vi "日志、报警信息存储 (子VI).vi"() -> ()   [LabVIEW 2016, in "德润DR803L超标留样.lvlib"]
panel:
  out "采样器状态":T1
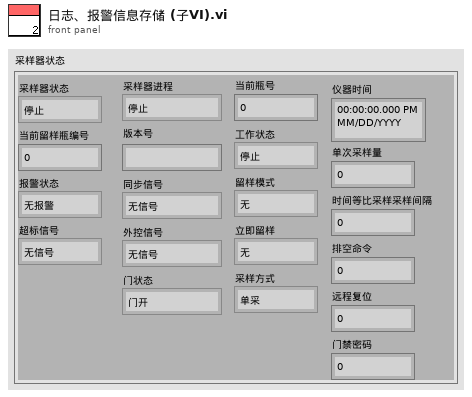
[diagram p1: front panel]
types:
  T1 = cluster{"采样器状态":enum16{"停止", "运行"}, "当前留样瓶编号":u16, "报警状态":enum16{"无报警", "缺水报警"}, "超标信号":enum16{"无信号", "超标信号"}, "采样器进程":enum16{"停止", "待机", "定位校正", "移除瓶盖", "采样瓶排空", "管路润洗", "管存", "进样", "瓶盖密封", "管路排空", "调整采样位置", "采样结束", "采样瓶润洗", "瓶润洗排空"}, "版本号":string, "同步信号":enum16{"无信号", "同步信号"}, "外控信号":enum16{"无信号", "外控信号"}, "门状态":enum16{"门开", "门关"}, "当前瓶号":u16, "工作状态":enum16{"停止", "采样中"}, "留样模式":enum16{"无", "定时留样", "时间等比例", "超标留样", "同步留样", "外控留样"}, "立即留样":enum16{"无", "远程留样"}, "采样方式":enum16{"单采", "双重"}, "仪器时间":timestamp, "单次采样量":u16, "时间等比采样采样间隔":u16, "排空命令":u16, "远程复位":u16, "门禁密码":u16}
  T2 = cluster{"时间标识":timestamp, "设备":string, "日志信息":string, "流程参数":string}
  T3 = cluster{"时间标识":timestamp, "设备":string, "日志信息":string}
  T4 = enum16{"停止", "待机", "定位校正", "移除瓶盖", "采样瓶排空", "管路润洗", "管存", "进样", "瓶盖密封", "管路排空", "调整采样位置", "采样结束", "采样瓶润洗", "瓶润洗排空"}
  T5 = enum16{"无", "定时留样", "时间等比例", "超标留样", "同步留样", "外控留样"}
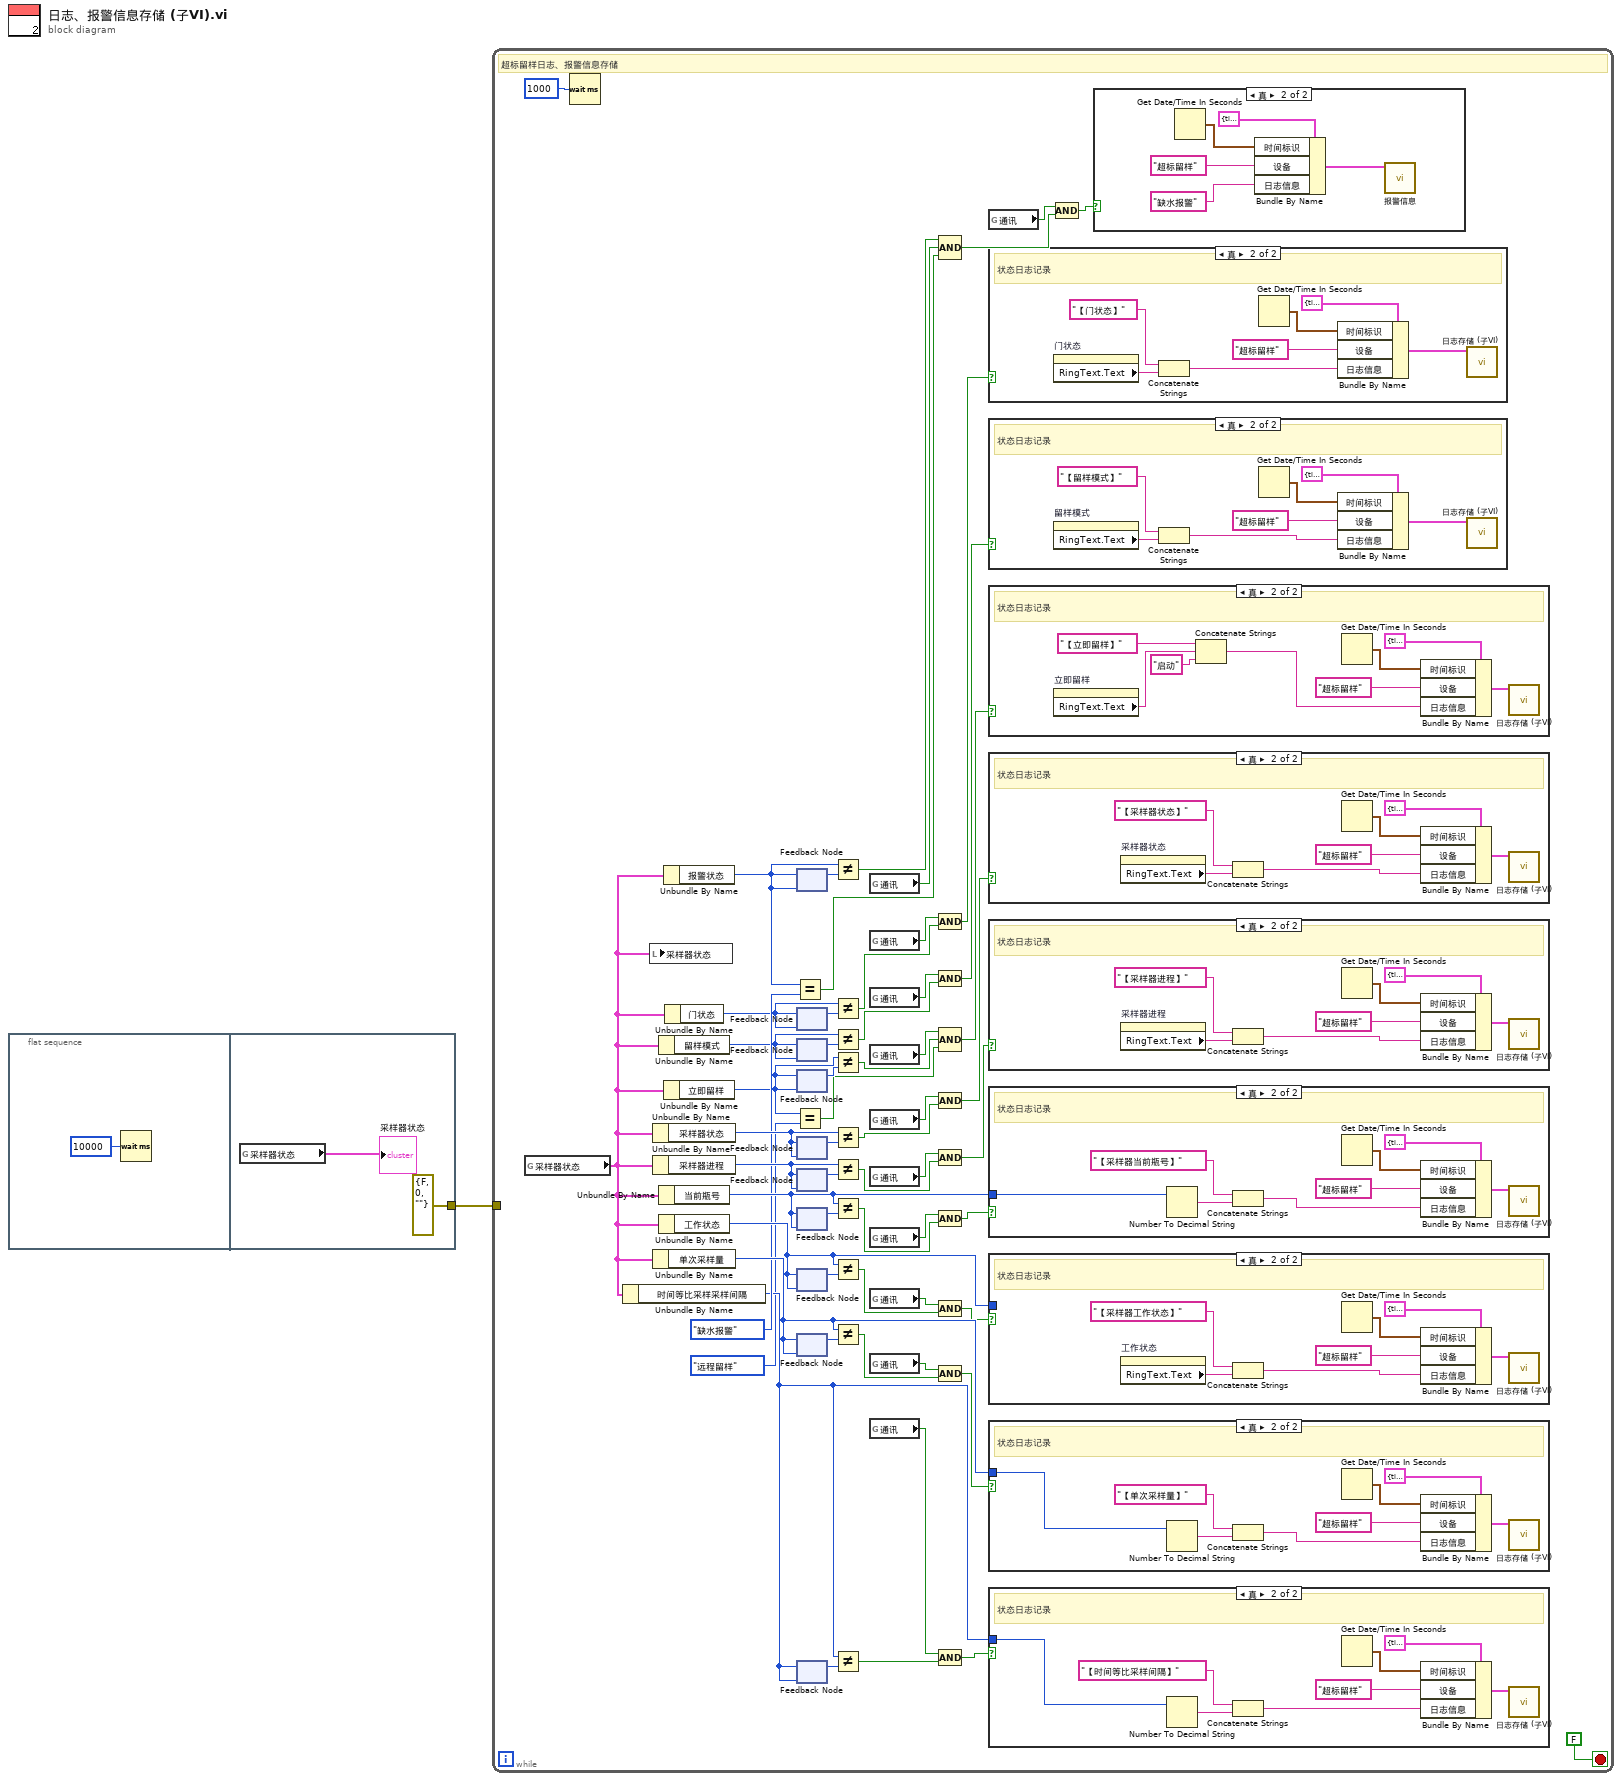
[diagram p0: block diagram]
diagram:
  n1 = flat-sequence {
    tunnel: [errorcluster {"status"=FALSE, "code"=0, "source"=""} ("错误常量")] -> w1
    frame #0 {
      n2 = Wait (ms)(milliseconds to wait=u32 10000 ("等待时间（毫秒）")) -> ()  [unwired: 1 out]
    }
    frame #1 {
      n3 = global read "超标留样全局.vi" "采样器状态"() -> (→"采样器状态":T1)
    }
  }
  n4 = while {
    tunnel: w1 -> [_]
    stop <- FALSE stop-if-true
    # "超标留样日志、报警信息存储"
    n5 = global read "超标留样全局.vi" "采样器状态"() -> (w5:T1)
    n6 = Wait (ms)(milliseconds to wait=u32 1000 ("等待时间（毫秒）")) -> ()  [unwired: 1 out]
    n7 = Unbundle By Name(w5) -> ("时间等比采样采样间隔"=w41:u16)
    n8 = local write "采样器状态"(w5) -> ()
    n9 = Unbundle By Name(w5) -> ("采样器状态"=w60:enum16{"停止", "运行"})
    n10 = Unbundle By Name(w5) -> ("采样器进程"=w59:T4)
    n11 = Unbundle By Name(w5) -> ("单次采样量"=w52:u16)
    n12 = Unbundle By Name(w5) -> ("留样模式"=w44:T5)
    n13 = Unbundle By Name(w5) -> ("当前瓶号"=w56:u16)
    n14 = Unbundle By Name(w5) -> ("工作状态"=w55:enum16{"停止", "采样中"})
    n15 = Unbundle By Name(w5) -> ("报警状态"=w47:enum16{"无报警", "缺水报警"})
    n16 = Unbundle By Name(w5) -> ("立即留样"=w40:enum16{"无", "远程留样"})
    n17 = Unbundle By Name(w5) -> ("门状态"=w45:enum16{"门开", "门关"})
    n18 = Equal?(x=w47, y=enum16{"无报警", "缺水报警"}."缺水报警" ("报警状态")) -> (x = y?=w35:bool)
    n19 = Equal?(x=w40, y=enum16{"无", "远程留样"}."远程留样" ("立即留样")) -> (x = y?=w8:bool)
    n20 = feedback #1(w47) -> (w50:enum16{"无报警", "缺水报警"})
    n21 = feedback-in #1(w47) -> ()
    n22 = feedback #2(w45) -> (w46:enum16{"门开", "门关"})
    n23 = feedback-in #2(w45) -> ()
    n24 = feedback #3(w44) -> (w43:T5)
    n25 = feedback-in #3(w44) -> ()
    n26 = feedback #4(w40) -> (w39:enum16{"无", "远程留样"})
    n27 = feedback-in #4(w40) -> ()
    n28 = feedback #5(w60) -> (w61:enum16{"停止", "运行"})
    n29 = feedback-in #5(w60) -> ()
    n30 = feedback #6(w59) -> (w58:T4)
    n31 = feedback-in #6(w59) -> ()
    n32 = feedback #7(w56) -> (w57:u16)
    n33 = feedback-in #7(w56) -> ()
    n34 = feedback #8(w55) -> (w54:enum16{"停止", "采样中"})
    n35 = feedback-in #8(w55) -> ()
    n36 = feedback #9(w52) -> (w53:u16)
    n37 = feedback-in #9(w52) -> ()
    n38 = feedback #10(w41) -> (w42:u16)
    n39 = feedback-in #10(w41) -> ()
    n40 = Not Equal?(x=w47, y=w50) -> (x != y?=w34:bool)
    n41 = Not Equal?(x=w45, y=w46) -> (x != y?=w31:bool)
    n42 = Not Equal?(x=w44, y=w43) -> (x != y?=w23:bool)
    n43 = Not Equal?(x=w40, y=w39) -> (x != y?=w7:bool)
    n44 = Not Equal?(x=w60, y=w61) -> (x != y?=w25:bool)
    n45 = Not Equal?(x=w59, y=w58) -> (x != y?=w26:bool)
    n46 = Not Equal?(x=w56, y=w57) -> (x != y?=w19:bool)
    n47 = Not Equal?(x=w55, y=w54) -> (x != y?=w17:bool)
    n48 = Not Equal?(x=w52, y=w53) -> (x != y?=w14:bool)
    n49 = Not Equal?(x=w41, y=w42) -> (x != y?=w10:bool)
    n50 = global read "超标留样全局.vi" "通讯"() -> (w37:bool)
    n51 = global read "超标留样全局.vi" "通讯"() -> (w33:bool)
    n52 = global read "超标留样全局.vi" "通讯"() -> (w30:bool)
    n53 = global read "超标留样全局.vi" "通讯"() -> (w9:bool)
    n54 = global read "超标留样全局.vi" "通讯"() -> (w29:bool)
    n55 = global read "超标留样全局.vi" "通讯"() -> (w28:bool)
    n56 = global read "超标留样全局.vi" "通讯"() -> (w21:bool)
    n57 = global read "超标留样全局.vi" "通讯"() -> (w18:bool)
    n58 = global read "超标留样全局.vi" "通讯"() -> (w15:bool)
    n59 = global read "超标留样全局.vi" "通讯"() -> (w12:bool)
    n60 = Compound Arithmetic op=AND ("复合运算")(w34, w37, w35) -> (w36:bool)
    n61 = Compound Arithmetic op=AND ("复合运算")(w33, w31) -> (w32:bool)
    n62 = Compound Arithmetic op=AND ("复合运算")(w30, w23) -> (w22:bool)
    n63 = Compound Arithmetic op=AND ("复合运算")(w9, w7, w8) -> (w6:bool)
    n64 = Compound Arithmetic op=AND ("复合运算")(w29, w25) -> (w24:bool)
    n65 = Compound Arithmetic op=AND ("复合运算")(w28, w26) -> (w27:bool)
    n66 = Compound Arithmetic op=AND ("复合运算")(w21, w19) -> (w20:bool)
    n67 = Compound Arithmetic op=AND ("复合运算")(w18, w17) -> (w16:bool)
    n68 = Compound Arithmetic op=AND ("复合运算")(w15, w14) -> (w13:bool)
    n69 = Compound Arithmetic op=AND ("复合运算")(w12, w10) -> (w11:bool)
    n70 = global read "超标留样全局.vi" "通讯"() -> (w51:bool)
    n71 = case shown="真" w32 {
      frame False {
      }
      frame True {
        # "状态日志记录"
        n72 = property on="门状态" class="Enum (严格)"() -> ("RingText.Text"=w87:string)  [unwired: 2 in, 2 out]
        n73 = Concatenate Strings("【门状态】" ("日志信息"), w87) -> (w93:string)
        n74 = Get Date/Time In Seconds() -> (seconds since 1Jan1904=w90:timestamp)
        n75 = Bundle By Name(cluster=T2 {"时间标识"=timestamp(0 s since 1904-01-01), "设备"="", "日志信息"="", "流程参数"=""} ("data in"), "时间标识"=w90, "设备"="超标留样", "日志信息"=w93) -> (w89:T2)
        n76 = call "日志存储 (子VI).vi"("data in"=w89) -> ()  [unwired: 11 in]
      }
    }
    n77 = case shown="真" w22 {
      frame False {
      }
      frame True {
        # "状态日志记录"
        n78 = property on="留样模式" class="Enum (严格)"() -> ("RingText.Text"=w80:string)  [unwired: 2 in, 2 out]
        n79 = Concatenate Strings("【留样模式】" ("日志信息"), w80) -> (w86:string)
        n80 = Get Date/Time In Seconds() -> (seconds since 1Jan1904=w83:timestamp)
        n81 = Bundle By Name(cluster=T2 {"时间标识"=timestamp(0 s since 1904-01-01), "设备"="", "日志信息"="", "流程参数"=""} ("data in"), "时间标识"=w83, "设备"="超标留样", "日志信息"=w86) -> (w82:T2)
        n82 = call "日志存储 (子VI).vi"("data in"=w82) -> ()  [unwired: 11 in]
      }
    }
    n83 = case shown="真" w6 {
      frame False {
      }
      frame True {
        # "状态日志记录"
        n84 = property on="立即留样" class="Enum (严格)"() -> ("RingText.Text"=w65:string)  [unwired: 2 in, 2 out]
        n85 = Concatenate Strings("【立即留样】" ("日志信息"), w65, "启动" ("字符串")) -> (w71:string)
        n86 = Get Date/Time In Seconds() -> (seconds since 1Jan1904=w68:timestamp)
        n87 = Bundle By Name(cluster=T2 {"时间标识"=timestamp(0 s since 1904-01-01), "设备"="", "日志信息"="", "流程参数"=""} ("data in"), "时间标识"=w68, "设备"="超标留样", "日志信息"=w71) -> (w67:T2)
        n88 = call "日志存储 (子VI).vi"("data in"=w67) -> ()  [unwired: 11 in]
      }
    }
    n89 = case shown="真" w24 {
      frame False {
      }
      frame True {
        # "状态日志记录"
        n90 = property on="采样器状态" class="Enum (严格)"() -> ("RingText.Text"=w129:string)  [unwired: 2 in, 2 out]
        n91 = Concatenate Strings("【采样器状态】" ("日志信息"), w129) -> (w135:string)
        n92 = Get Date/Time In Seconds() -> (seconds since 1Jan1904=w132:timestamp)
        n93 = Bundle By Name(cluster=T2 {"时间标识"=timestamp(0 s since 1904-01-01), "设备"="", "日志信息"="", "流程参数"=""} ("data in"), "时间标识"=w132, "设备"="超标留样", "日志信息"=w135) -> (w131:T2)
        n94 = call "日志存储 (子VI).vi"("data in"=w131) -> ()  [unwired: 11 in]
      }
    }
    n95 = case shown="真" w27 {
      frame False {
      }
      frame True {
        # "状态日志记录"
        n96 = property on="采样器进程" class="Enum (严格)"() -> ("RingText.Text"=w122:string)  [unwired: 2 in, 2 out]
        n97 = Concatenate Strings("【采样器进程】" ("日志信息"), w122) -> (w128:string)
        n98 = Get Date/Time In Seconds() -> (seconds since 1Jan1904=w125:timestamp)
        n99 = Bundle By Name(cluster=T2 {"时间标识"=timestamp(0 s since 1904-01-01), "设备"="", "日志信息"="", "流程参数"=""} ("data in"), "时间标识"=w125, "设备"="超标留样", "日志信息"=w128) -> (w124:T2)
        n100 = call "日志存储 (子VI).vi"("data in"=w124) -> ()  [unwired: 11 in]
      }
    }
    n101 = case shown="真" w20 {
      tunnel: w56 -> [_ w115]
      frame False {
      }
      frame True {
        # "状态日志记录"
        n102 = Number To Decimal String(number=w115) -> (decimal integer string=w114:string)  [unwired: 1 in]
        n103 = Concatenate Strings("【采样器当前瓶号】" ("日志信息"), w114) -> (w121:string)
        n104 = Get Date/Time In Seconds() -> (seconds since 1Jan1904=w118:timestamp)
        n105 = Bundle By Name(cluster=T2 {"时间标识"=timestamp(0 s since 1904-01-01), "设备"="", "日志信息"="", "流程参数"=""} ("data in"), "时间标识"=w118, "设备"="超标留样", "日志信息"=w121) -> (w117:T2)
        n106 = call "日志存储 (子VI).vi"("data in"=w117) -> ()  [unwired: 11 in]
      }
    }
    n107 = case shown="真" w16 {
      tunnel: w55 -> [_ _]
      frame False {
      }
      frame True {
        # "状态日志记录"
        n108 = property on="工作状态" class="Enum (严格)"() -> ("RingText.Text"=w107:string)  [unwired: 2 in, 2 out]
        n109 = Concatenate Strings("【采样器工作状态】" ("日志信息"), w107) -> (w113:string)
        n110 = Get Date/Time In Seconds() -> (seconds since 1Jan1904=w110:timestamp)
        n111 = Bundle By Name(cluster=T2 {"时间标识"=timestamp(0 s since 1904-01-01), "设备"="", "日志信息"="", "流程参数"=""} ("data in"), "时间标识"=w110, "设备"="超标留样", "日志信息"=w113) -> (w109:T2)
        n112 = call "日志存储 (子VI).vi"("data in"=w109) -> ()  [unwired: 11 in]
      }
    }
    n113 = case shown="真" w13 {
      tunnel: w52 -> [_ w100]
      frame False {
      }
      frame True {
        # "状态日志记录"
        n114 = Number To Decimal String(number=w100) -> (decimal integer string=w99:string)  [unwired: 1 in]
        n115 = Concatenate Strings("【单次采样量】" ("日志信息"), w99) -> (w106:string)
        n116 = Get Date/Time In Seconds() -> (seconds since 1Jan1904=w103:timestamp)
        n117 = Bundle By Name(cluster=T2 {"时间标识"=timestamp(0 s since 1904-01-01), "设备"="", "日志信息"="", "流程参数"=""} ("data in"), "时间标识"=w103, "设备"="超标留样", "日志信息"=w106) -> (w102:T2)
        n118 = call "日志存储 (子VI).vi"("data in"=w102) -> ()  [unwired: 11 in]
      }
    }
    n119 = case shown="真" w11 {
      tunnel: w41 -> [_ w73]
      frame False {
      }
      frame True {
        # "状态日志记录"
        n120 = Number To Decimal String(number=w73) -> (decimal integer string=w72:string)  [unwired: 1 in]
        n121 = Concatenate Strings("【时间等比采样间隔】" ("日志信息"), w72) -> (w79:string)
        n122 = Get Date/Time In Seconds() -> (seconds since 1Jan1904=w76:timestamp)
        n123 = Bundle By Name(cluster=T2 {"时间标识"=timestamp(0 s since 1904-01-01), "设备"="", "日志信息"="", "流程参数"=""} ("data in"), "时间标识"=w76, "设备"="超标留样", "日志信息"=w79) -> (w75:T2)
        n124 = call "日志存储 (子VI).vi"("data in"=w75) -> ()  [unwired: 11 in]
      }
    }
    n125 = Compound Arithmetic op=AND ("复合运算")(w51, w36) -> (w49:bool)
    n126 = case shown="真" w49 {
      frame False {
      }
      frame True {
        n127 = Get Date/Time In Seconds() -> (seconds since 1Jan1904=w98:timestamp)
        n128 = Bundle By Name(cluster=T3 {"时间标识"=timestamp(0 s since 1904-01-01), "设备"="", "日志信息"=""} ("data in"), "时间标识"=w98, "设备"="超标留样", "日志信息"="缺水报警") -> (w94:T3)
        n129 = call "报警信息.vi"("data in"=w94) -> ()  [unwired: 10 in, 1 out]
      }
    }
  }
